vi "destroy.vi"(0 "datasource_pdf in":refnum<class "datasource_pdf.lvclass">, 11 "error in (no error)":errorcluster) -> (4 "datasource_pdf out":refnum<class "datasource_pdf.lvclass">, 15 "error out":errorcluster)   [LabVIEW 2020, in "datasource_pdf.lvclass"]
uses:
  datasource_pdf.lvclass
  datasource_pdf.lvclass/datasource_pdf.ctl
  models/abstract_llm_base/abstract_llm_base.lvclass
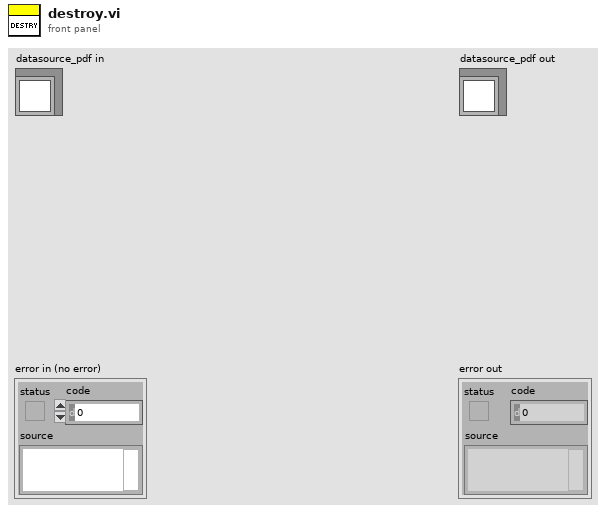
[diagram p1: front panel]
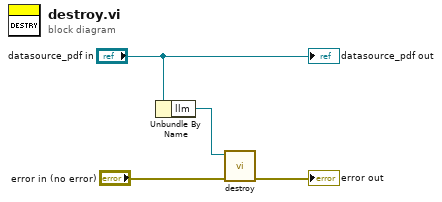
[diagram p0: block diagram]
diagram:
  n1 = Unbundle By Name("datasource_pdf in") -> ("llm"=w1:refnum<class "abstract_llm_base.lvclass">)
  n2 = call-dynamic "destroy.vi"("error in (no error)"="error in (no error)", "abstract_llm_base in"=w1) -> ("error out"=→"error out":errorcluster)  [unwired: 8 in, 1 out]
  "datasource_pdf out" <- "datasource_pdf in"
